vi "temp.vi"() -> ()   [LabVIEW 2014]
uses:
  Position.lvclass
panel:
  in  "Anchor 2 X":dbl=60.0
  in  "Anchor 1 X":dbl=5.0
  in  "Anchor 1 Y":dbl=30.0
  in  "Anchor 2 Y":dbl=56.0
  in  "Anchor 3 X":dbl=115.0
  in  "Anchor 3 Y":dbl=30.0
  out "Output":string[][](array[string])
  in  "Intersections Array":T1(array[cluster])
  out "Iteration":i32
  out "Rest array":string[][](array[string])
  out "x1 1":dbl
  out "y1 1":dbl
  out "x2 1":dbl
  out "y2 1":dbl
  out "Flat Batch Array":string[](array[string])
  out "R Anchor 1":dbl
  out "R Anchor 2":dbl
  out "R Anchor 3":dbl
  out "x1 3":dbl
  out "x1 2":dbl
  out "y1 2":dbl
  out "x2 2":dbl
  out "y2 2":dbl
  out "y1 3":dbl
  out "x2 3":dbl
  out "y2 3":dbl
  out "Batch":string[][](array[string])
  out "time":string[](array[string])
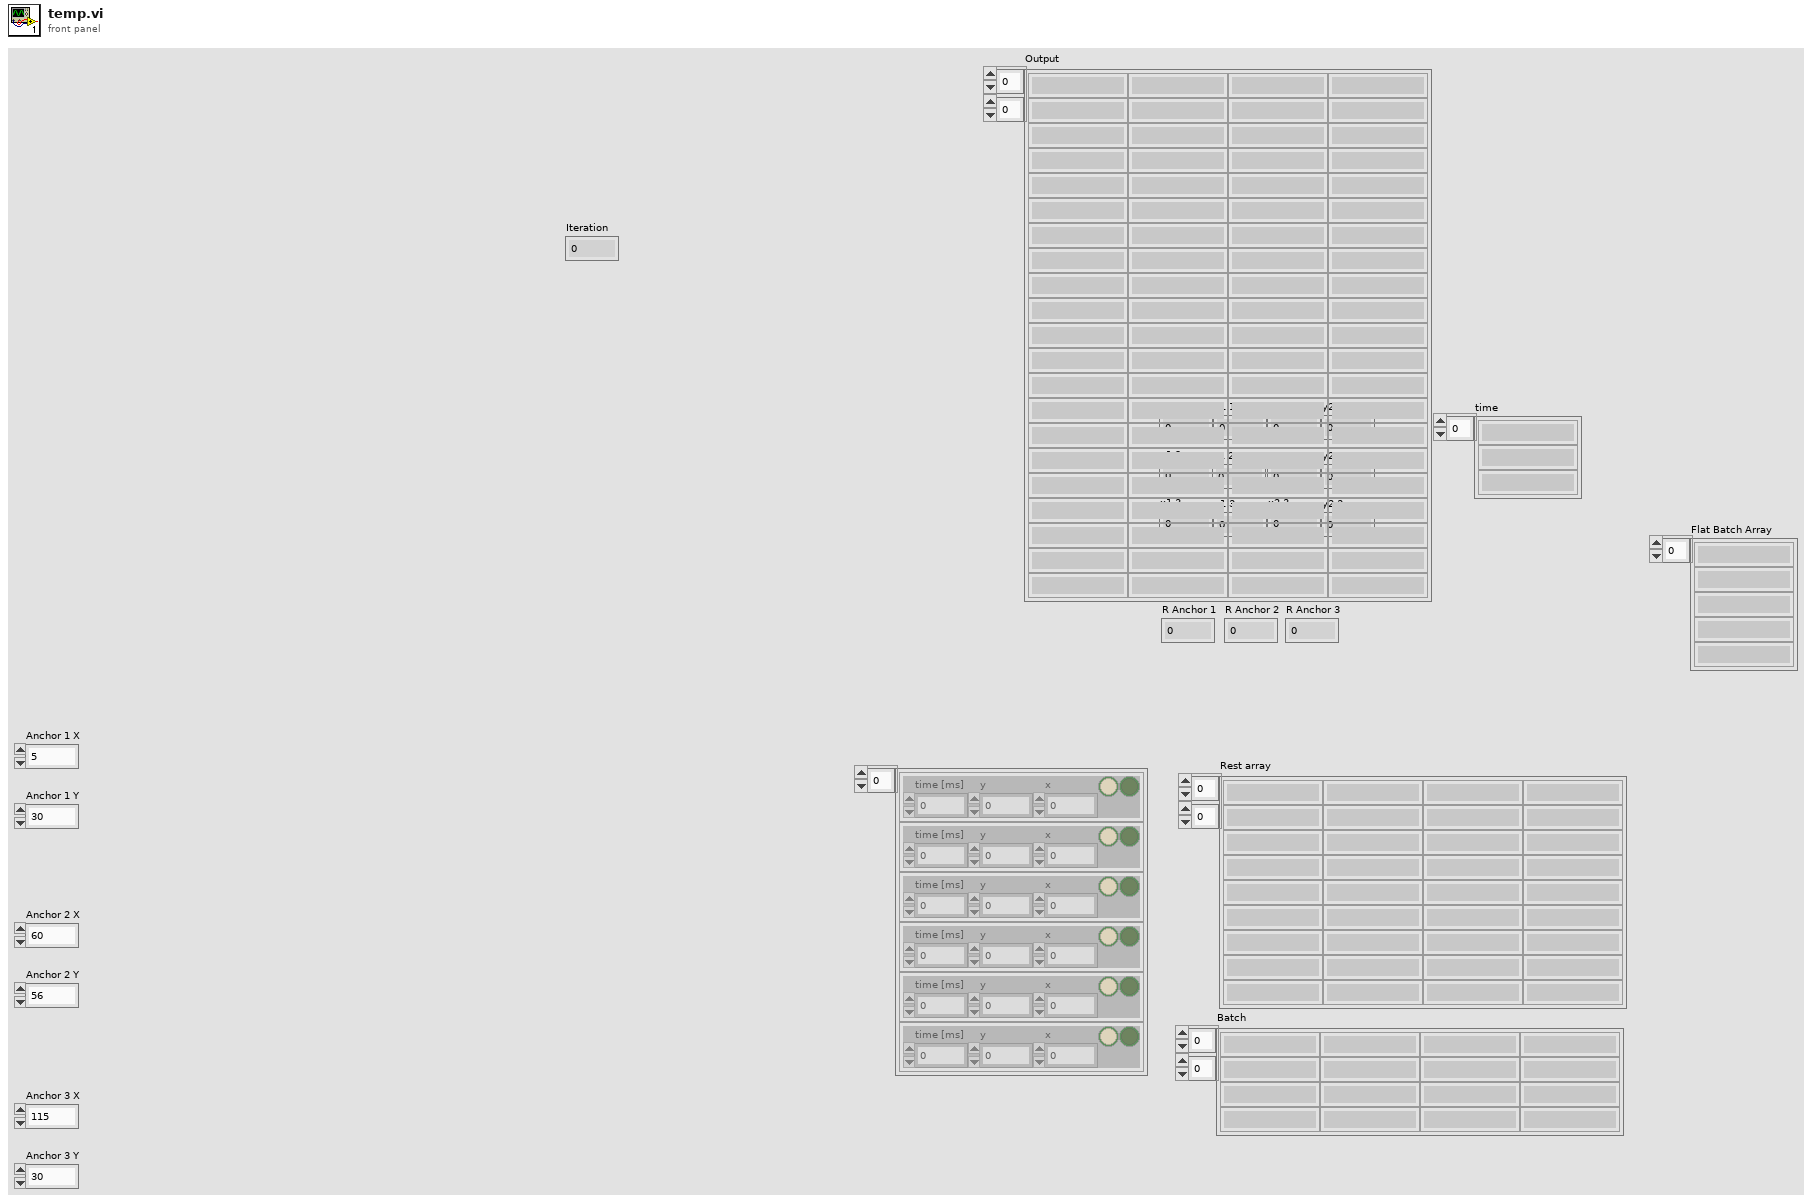
[diagram p1: front panel]
types:
  T1 = cluster{"time [ms]":dbl, "y":dbl, "x":dbl, "Fout":bool, "Goed":bool}[]
  T2 = cluster{"Time [ms]":dbl, "y":dbl, "x":dbl, "Fout":bool, "Goed":bool}[]
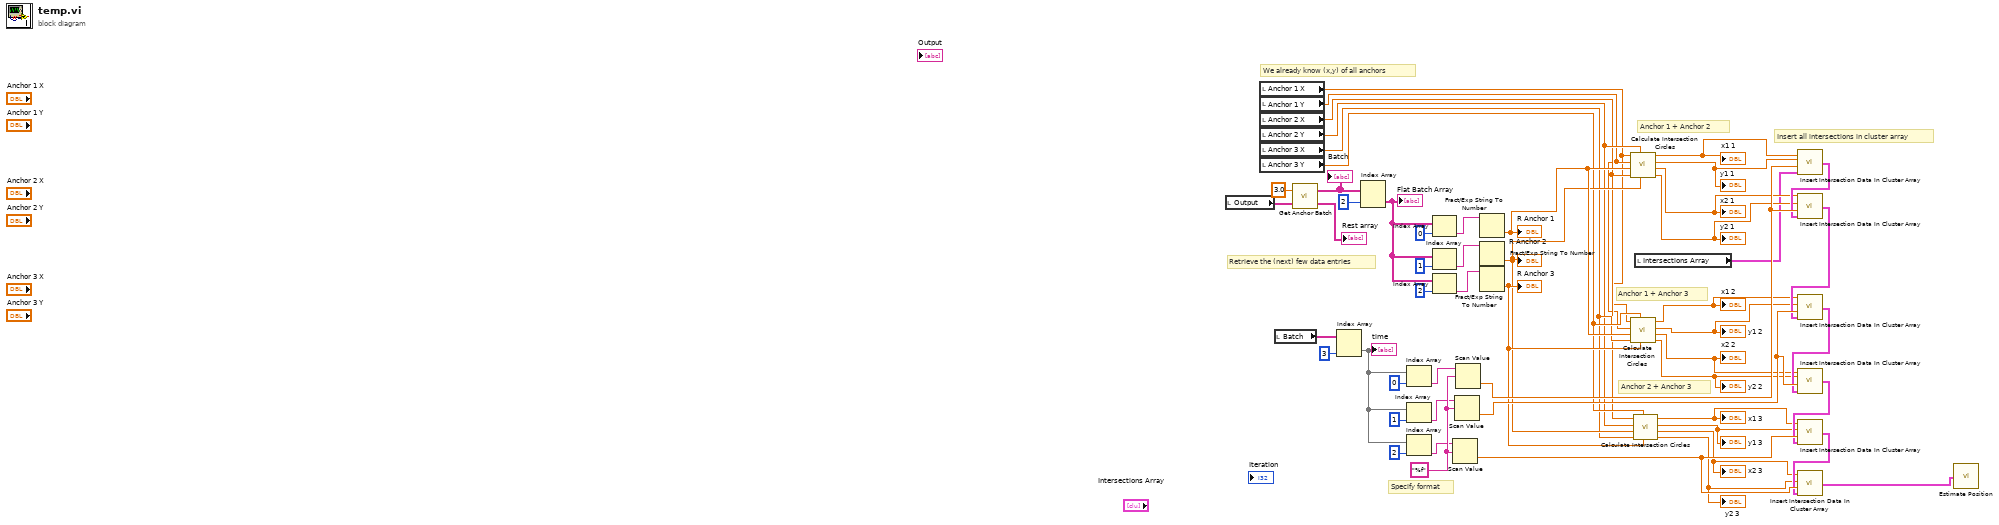
[diagram p0: block diagram]
diagram:
  w51 = "%f" ("format string")
  # "Insert all intersections in cluster array"
  # "Specify format"
  # "Retrieve the (next) few data entries"
  # "Anchor 2 + Anchor 3"
  # "Anchor 1 + Anchor 3"
  # "Anchor 1 + Anchor 2"
  # "We already know (x,y) of all anchors"
  n1 = local read "Output"() -> (w2:string[][])
  n2 = local read "Anchor 1 X"() -> (w13:dbl)
  n3 = local read "Anchor 1 Y"() -> (w14:dbl)
  n4 = local read "Anchor 2 X"() -> (w15:dbl)
  n5 = local read "Anchor 2 Y"() -> (w16:dbl)
  n6 = local read "Anchor 3 X"() -> (w17:dbl)
  n7 = local read "Anchor 3 Y"() -> (w18:dbl)
  n8 = local read "Batch"() -> (w21:string[][])
  n9 = call "Get Anchor Batch.vi"("Input Array"=w2, "Batch size"=3.0) -> ("Rest array"=→"Rest array":string[][], "Batch array"=w4:string[][])
  "Batch" <- w4
  n10 = Index Array(array=w21, index (col)=3 ("disabled index (col)")) -> (element=w23:string[])  [unwired: 1 in]
  "time" <- w23
  n11 = Index Array "Index Array"(array=w4, index (col)=2 ("index (row)")) -> (element=w8:string[])  [unwired: 1 in]
  "Flat Batch Array" <- w8
  n12 = Index Array(array=w23, index=0) -> (element=w50:string)
  n13 = Index Array(array=w23, index=1) -> (element=w48:string)
  n14 = Index Array(array=w23, index=2) -> (element=w45:string)
  n15 = Index Array(array=w8, index=0) -> (element=w7:string)
  n16 = Index Array(array=w8, index=1) -> (element=w11:string)
  n17 = Index Array(array=w8, index=2) -> (element=w12:string)
  n18 = Scan Value(string=w45, format string=w51) -> (value=w46:dbl)  [unwired: 1 in, 1 out]
  n19 = Scan Value(string=w48, format string=w51) -> (value=w47:dbl)  [unwired: 1 in, 1 out]
  n20 = Scan Value(string=w50, format string=w51) -> (value=w49:dbl)  [unwired: 1 in, 1 out]
  n21 = Fract/Exp String To Number(string=w7) -> (number=w52:dbl)  [unwired: 3 in, 1 out]
  "R Anchor 1" <- w52
  n22 = Fract/Exp String To Number(string=w11) -> (number=w19:dbl)  [unwired: 3 in, 1 out]
  "R Anchor 2" <- w19
  n23 = Fract/Exp String To Number(string=w12) -> (number=w20:dbl)  [unwired: 3 in, 1 out]
  "R Anchor 3" <- w20
  n24 = call "Calculate Intersection Circles.vi"("r2"=w19, "d"=w16, "c"=w15, "r1"=w52, "b"=w14, "a"=w13) -> ("y2"=w31:dbl, "x2"=w30:dbl, "y1"=w28:dbl, "x1"=w27:dbl)
  "x1 1" <- w27
  "y1 1" <- w28
  "x2 1" <- w30
  "y2 1" <- w31
  n25 = call "Calculate Intersection Circles.vi"("r2"=w20, "d"=w18, "c"=w17, "r1"=w52, "b"=w14, "a"=w13) -> ("y2"=w35:dbl, "x2"=w34:dbl, "y1"=w33:dbl, "x1"=w32:dbl)
  "x1 2" <- w32
  "y1 2" <- w33
  "x2 2" <- w34
  "y2 2" <- w35
  n26 = call "Calculate Intersection Circles.vi"("r2"=w20, "d"=w18, "c"=w17, "r1"=w19, "b"=w16, "a"=w15) -> ("y2"=w39:dbl, "x2"=w38:dbl, "y1"=w37:dbl, "x1"=w36:dbl)
  "x1 3" <- w36
  "y1 3" <- w37
  "x2 3" <- w38
  "y2 3" <- w39
  n27 = local read "Intersections Array"() -> (w29:T1)
  n28 = call "Insert Intersection Data In Cluster Array.vi"("Cluster Array"=w29, "Time"=w49, "Y"=w28, "X"=w27) -> ("Intersections"=w40:T2)
  n29 = call "Insert Intersection Data In Cluster Array.vi"("Cluster Array"=w40, "Time"=w49, "Y"=w31, "X"=w30) -> ("Intersections"=w41:T2)
  n30 = call "Insert Intersection Data In Cluster Array.vi"("Cluster Array"=w41, "Time"=w47, "Y"=w33, "X"=w32) -> ("Intersections"=w42:T2)
  n31 = call "Insert Intersection Data In Cluster Array.vi"("Cluster Array"=w42, "Time"=w47, "Y"=w35, "X"=w34) -> ("Intersections"=w43:T2)
  n32 = call "Insert Intersection Data In Cluster Array.vi"("Cluster Array"=w43, "Time"=w46, "Y"=w37, "X"=w36) -> ("Intersections"=w44:T2)
  n33 = call "Insert Intersection Data In Cluster Array.vi"("Cluster Array"=w44, "Time"=w46, "Y"=w39, "X"=w38) -> ("Intersections"=w53:T2)
  n34 = call "Estimate Position.vi"("Intersections"=w53) -> ()  [unwired: 2 out]
